vi "Read Hallway.vi"(8 "error in (no error)":errorcluster, 11 "State in":refnum<class "State.lvclass">) -> (0 "error out":errorcluster, 2 "Hallway":string[](array[string]), 3 "State out":refnum<class "State.lvclass">)   [LabVIEW 2019, in "23.lvlib" / "State.lvclass"]
uses:
  State.lvclass
  C:/Users/craig.walker/Documents/GitHub/lv2019-LRU-Cache/LRU Node/LRU Node.lvclass
  lv2019-LRU-Cache/LRU Node/LRU Node.lvclass/LRU Node.ctl
  State Key/State Key.lvclass
  lv2019-LRU-Cache/LRU Node/LRU Node.lvclass
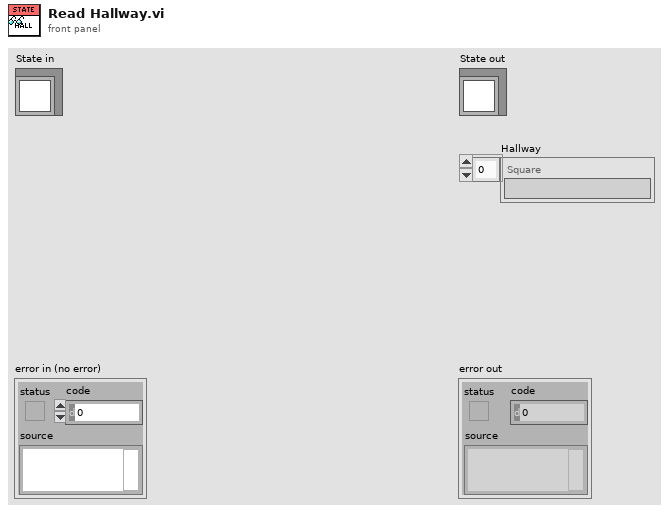
[diagram p1: front panel]
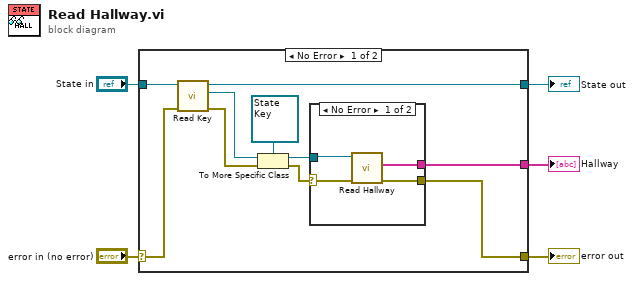
[diagram p0: block diagram]
diagram:
  n1 = case shown="No Error" "error in (no error)" {
    selector: "error in (no error)" -> [w7 w20]
    tunnel: [w6 w20] -> w4
    tunnel: [w15 w21] -> w2
    tunnel: "State in" -> [w14 w21]
    tunnel: [w8 _] -> w1
    frame No Error {
      n2 = call "Read Key.vi"("error in (no error)"=w7, "LRU Node in"=w14) -> ("error out"=w9:errorcluster, "Key"=w13:refnum<class>, "LRU Node out"=w15:refnum<class "State.lvclass">)  [unwired: 7 in]
      n3 = To More Specific Class(target class=refnum<class "State Key.lvclass"> refnum ("23.lvlib:State Key.lvclass"), reference=w13, error in=w9) -> (specific class reference=w10:refnum<class "State Key.lvclass">, error out=w11:errorcluster)
      n4 = case shown="No Error" w11 {
        selector: w11 -> [w18 _]
        tunnel: w10 -> [w19 _]
        tunnel: [w17 _] -> w8
        tunnel: [w16 _] -> w6
        frame No Error {
          n5 = call-dynamic "Read Hallway.vi"("error in (no error)"=w18, "State Key in"=w19) -> ("error out"=w16:errorcluster, "Hallway"=w17:string[])  [unwired: 7 in, 1 out]
        }
        frame Error {
        }
      }
    }
    frame Error {
    }
  }
  "error out" <- w4
  "State out" <- w2
  "Hallway" <- w1
